vi "Nastajmer3.vi"(8 "error in (no error)":errorcluster, 10 "Time Target":dbl, 11 "Enum":T2) -> (0 "error out":errorcluster, 2 "Timer Data Out":T1, 3 "Status":cluster{"Running":bool, "Done":bool})   [LabVIEW 2014]
uses:
  Control Timer3.ctl
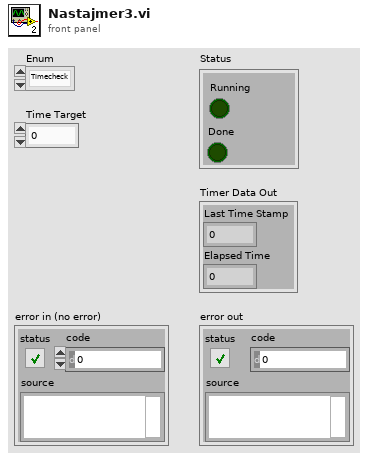
[diagram p1: front panel]
types:
  T1 = cluster{"Last Time Stamp":dbl, "Elapsed Time":dbl}
  T2 = typedef "Control Timer3.ctl" = enum16{"Timecheck", "Reset"}
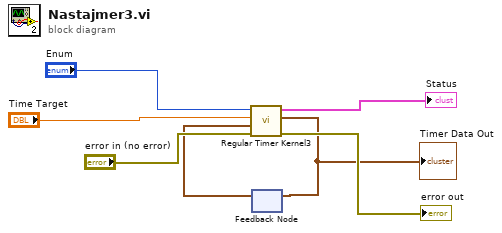
[diagram p0: block diagram]
diagram:
  n1 = feedback #1() -> (w2:T1)  [unwired: 1 in]
  n2 = call "Regular Timer Kernel3.vi"("error in"="error in (no error)", "Timer Data In"=w2, "Time Target"="Time Target", "Enum"="Enum") -> ("error out"=→"error out":errorcluster, "Timer Data Out"=w1:T1, "Status"=→"Status":cluster{"Running":bool, "Done":bool})  [unwired: 5 in]
  "Timer Data Out" <- w1
  n3 = feedback-in #1(w1) -> ()
